vi "AML Error Control.vi"(8 "input cluster":errorcluster, 11 "Error count":i32) -> (0 "error out":errorcluster, 2 "State out":string, 3 "Error count out":i32)   [LabVIEW 2019, in "PGC2D.lvlib"]
uses:
  PGC2D.lvlib
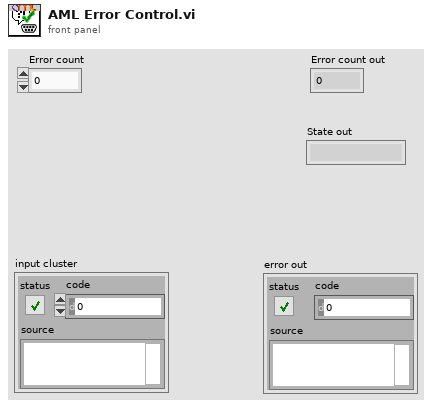
[diagram p1: front panel]
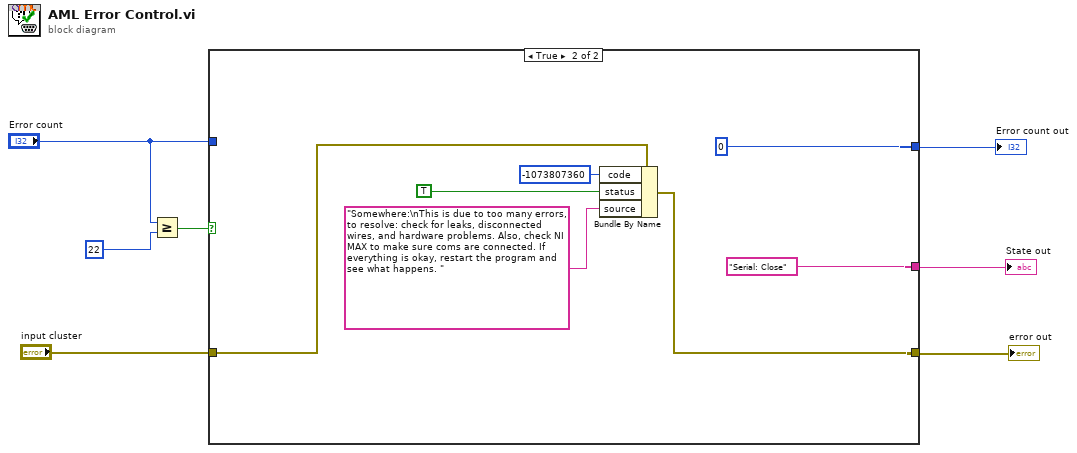
[diagram p0: block diagram]
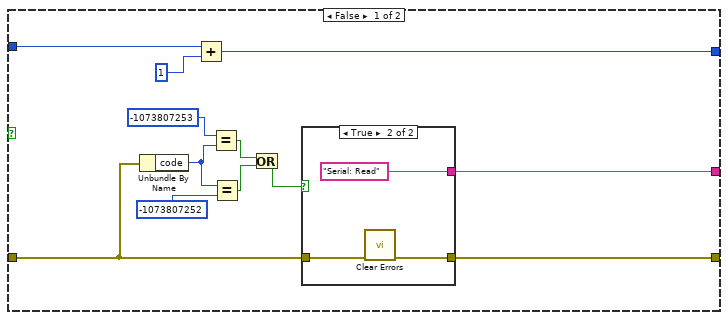
[diagram p2: hidden frame]
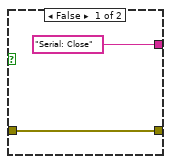
[diagram p3: hidden frame]
diagram:
  n1 = Greater Or Equal?(x="Error count", y=22) -> (x >= y?=w5:bool)
  n2 = case shown="True" w5 {
    tunnel: "input cluster" -> [w13 w29]
    tunnel: [w12 w26] -> w6
    tunnel: "Error count" -> [w11 _]
    tunnel: [w9 0] -> w1
    tunnel: [w8 "Serial: Close"] -> w2
    frame False {
      n3 = Unbundle By Name(w13) -> ("code"=w17:i32)
      n4 = Add(x=w11, y=1) -> (x+y=w9:i32)
      n5 = Equal?(x=-1073807253 ("specific error code to clear (0: all)"), y=w17) -> (x = y?=w16:bool)
      n6 = Equal?(x=w17, y=-1073807252 ("specific error code to clear (0: all)")) -> (x = y?=w15:bool)
      n7 = Or(x=w16, y=w15) -> (x .or. y?=w14:bool)
      n8 = case shown="True" w14 {
        tunnel: ["Serial: Close" "Serial: Read"] -> w8
        tunnel: w13 -> [w20 w23]
        tunnel: [w20 w22] -> w12
        frame False {
        }
        frame True {
          n9 = call <vilib>:"Clear Errors.vi"("error in (no error)"=w23) -> ("error out"=w22:errorcluster)  [unwired: 5 in, 1 out]
        }
      }
    }
    frame True {
      n10 = Bundle By Name(cluster=w29, "code"=-1073807360, "status"=TRUE, "source"="Somewhere:\nThis is due to too many errors, to resolve: check for leaks, disconnected wires, and hardware problems. Also, check NI MAX to make sure coms are connected. If everything is okay, restart the program and see what happens. ") -> (w26:errorcluster)
    }
  }
  "error out" <- w6
  "State out" <- w2
  "Error count out" <- w1
